vi "Update center freq.vi"(9 "error in (no error)":errorcluster) -> (1 "error out":errorcluster)   [LabVIEW 2017]
uses:
  Typedefs/HW config states enum.ctl
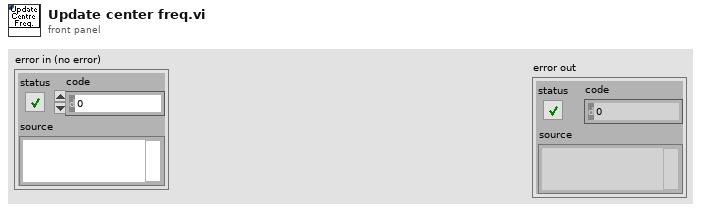
[diagram p1: front panel]
types:
  T1 = typedef "HW config states enum.ctl" = enum16{"Load from file", "Save to file", "Write all", "Read all", "Write XY stage settings", "Write DAQ FPGA settings", "Write Control FPGA settings", "Write Phys Channels", "Clear", "Compare from file"}
  T2 = typedef "System Configuration.ctl" = cluster{"Laser wavelength (nm)":dbl, "DAQ FPGA System":T3, "Control system":T5}
  T3 = typedef "DAQ FPGA system config.ctl" = cluster{"Clock Freq (MHz) ":dbl, "Samples Wait after Trigger":u16, "AOD fill":u16, "StartupDelay":i32, "Slip Cycle (clock cycles)":u32, "Add Cycle":bool, "Ref":T4}
  T4 = typedef "FPGA Ref.ctl" = refnum<k20>
  T5 = typedef "CTRL system config.ctl" = cluster{"AOD 1 Amplitude":i16, "AOD 2 Amplitude":i16, "AOD 3 Amplitude":i16, "AOD 4 Amplitude":i16, "AOD 5 Amplitude":i16, "AOD 6 Amplitude":i16, "T0 (ns)":dbl, "Ta (ns)":dbl, "Data Time Interval (ns)":dbl, "Ctrl FPGA Clock (MHz)":dbl, "Ethernet opened":bool}
  T6 = typedef "AOL_Globals.ctl" = cluster{"Imaging Protocol":T7, "Number of POI":u16, "Number of Miniscans":u16, "Number of Trials":u16, "Number of Cycles ":u64, "# Averaged Frames":u16, "Laser power (%)":u8, "Pockels":dbl, "Acquisition Length (sec)":dbl, "Fill time (us)":dbl, "POI Dwell time (us)":dbl, "Miniscan Dwell time per pixel (us)":dbl, "PMT 1":dbl, "PMT 2":dbl, "Back Apperture":dbl, "Frame Size":T8, "Center Frequency":dbl, "Field of View":dbl, "DwellTime (us)":dbl, "Wavelength (nm)":dbl, "Zoom":dbl, "AOL Z":dbl, "AOL Mode":T9, "GridXY":dbl, "GridZ":dbl, "TriggerPeriod (sec)":dbl, "Number of Pixels in Miniscan":u16, "Experiment folder path":path, "X centre":dbl, "Y centre":dbl, "Angle (degrees)":dbl, "Plane Mode":T10, "Threshold":u16[], "Regenerate Chirps":bool, "Rectangle ROI length (pixels)":u16, "Rectangle ROI height (pixels)":u16, "AOD fill":u16, "StartupDelay":i32, "Samples Wait after Trigger":u16, "Slip Cycle":u32, "Add Cycle":bool}
  T7 = typedef "Imaging Protocols enum.ctl" = enum16{"AOL Z-Stack", "Motor Z Stack", "Functional Acquisition", "Single Plane Acquisition", "Volume Acquisition", "Live Imaging", "Live Plane Imaging", "Live Volume Imaging"}
  T8 = typedef "Frame Size.ctl" = u16
  T9 = typedef "AOL modes.ctl" = enum16{"Raster", "Structural", "Pointing", "Mini Scan", "Alignment"}
  T10 = typedef "Plane Mode.ctl" = u16
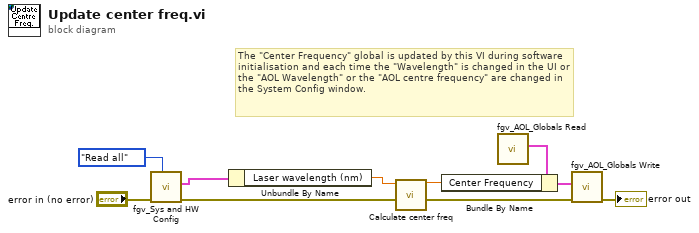
[diagram p0: block diagram]
diagram:
  # "The \"Center Frequency\" global is updated by this VI during software initialisation and each time the \"Wavelength\" is changed in the UI or the \"AOL Wavelength\" or the \"AOL centre frequency\" are changed in the System Config window."
  n1 = call "fgv_Sys and HW Config.vi"("Function"=HW_config_states_enum."Read all", "error in (no error)"="error in (no error)") -> ("error out"=w2:errorcluster, "System Config OUT"=w1:T2)  [unwired: 7 in, 1 out]
  n2 = Unbundle By Name(w1) -> ("Laser wavelength (nm)"=w8:dbl)
  n3 = call "Calculate center freq.vi"("error in (no error)"=w2, "UI Wavelength"=w8) -> ("error out"=w5:errorcluster, "Centre frequency (MHz)"=w6:dbl)  [unwired: 8 in]
  n4 = call "fgv_AOL_Globals Read.vi"() -> ("AOL_Globals"=w9:T6)  [unwired: 9 in, 2 out]
  n5 = Bundle By Name(cluster=w9, "Center Frequency"=w6) -> (w10:T6)
  n6 = call "fgv_AOL_Globals Write.vi"("error in (no error)"=w5, "AOL_Globals"=w10) -> ("error out"=→"error out":errorcluster)  [unwired: 9 in]
